vi "main_nova.vi"() -> ()   [LabVIEW 2020]
panel:
  out "Log":string
  in  "MoveJ 2":bool
  out "Error Log":string
  out "error out 3":errorcluster
  in  "MoveL":bool
  out "DigitalOutput":u8[](array[numeric])
  out "DigitalInput":u8[](array[numeric])
  out "Current SpeedFactor":dbl
  out "error out 2":errorcluster
  in  "Digital Outputs Index:":i32=1 min=1 max=16 step=1
  in  "GetErrorID":bool
  out "x value":string
  out "y value":string
  out "z value":string
  out "rx value":string
  out "ry value":string
  out "rz value":string
  out "j6 value":string
  out "j5 value":string
  out "j4 value":string
  out "j3 value":string
  out "j2 value":string
  out "j1 value":string
  in  "rz-":bool
  in  "ry-":bool
  in  "rx-":bool
  in  "z-":bool
  in  "y-":bool
  in  "x-":bool
  in  "rz+":bool
  in  "ry+":bool
  in  "rx+":bool
  in  "z+":bool
  in  "y+":bool
  in  "x+":bool
  in  "j6":dbl
  in  "j5":dbl
  in  "j4":dbl
  in  "j3":dbl
  in  "j2":dbl
  in  "j1":dbl
  in  "Set IO confrim":bool
  in  "Status":string(combo)="1"
  in  "Feedback Port":string="30004"
  in  "Dashboard Port":string="29999"
  in  "IP Address":string="192.168.5.1"
  in  "stop get state":bool
  out "state error out 2":errorcluster
  out "Robot mode":T1(ring)
  out "speed set string":string
  in  "j6-":bool
  in  "j5-":bool
  in  "j4-":bool
  in  "j3-":bool
  in  "j2-":bool
  in  "j1-":bool
  in  "j6+":bool
  in  "j5+":bool
  in  "j4+":bool
  in  "j3+":bool
  in  "j2+":bool
  in  "j1+":bool
  in  "stop connect":bool
  in  "Start trace":bool
  in  "tracePath":string
  in  "Stop move":bool
  in  "MoveJ":bool
  in  "rz":dbl
  in  "ry":dbl
  in  "rx":dbl
  in  "z":dbl
  in  "y":dbl
  in  "x":dbl
  in  "Speed confrim":bool
  in  "Speed Ratio":dbl=50.0
  in  "ClearError":bool
  in  "Enable Robot":bool
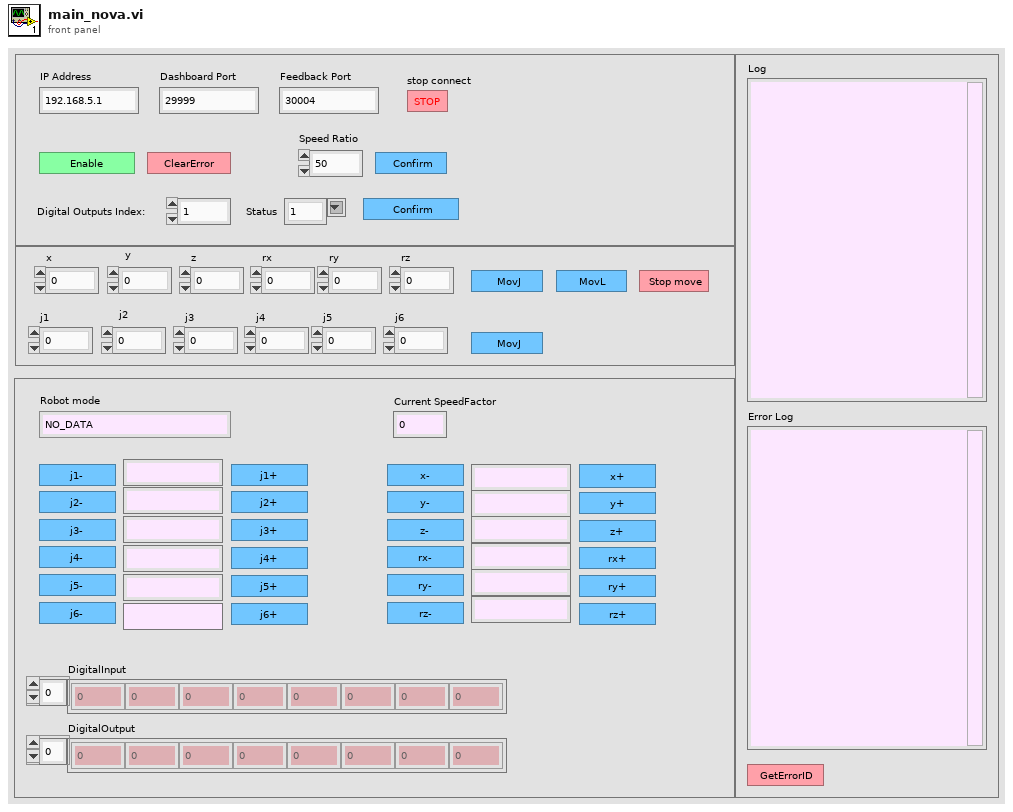
[diagram p1: front panel]
types:
  T1 = enum16{"NO_DATA", "ROBOT_MODE_INIT", "ROBOT_MODE_BRAKE_OPEN", "ROBOT_MODE_POWEROFF", "ROBOT_MODE_DISABLED", "ROBOT_MODE_ENABLE", "ROBOT_MODE_BACKDRIVE", "ROBOT_MODE_RUNNING", "ROBOT_MODE_SINGLE_MOVE", "ROBOT_MODE_ERROR", "ROBOT_MODE_PAUSE", "ROBOT_MODE_COLLISION"}
  T2 = enum16{"Standard", "Buffered", "CRLF", "Immediate"}
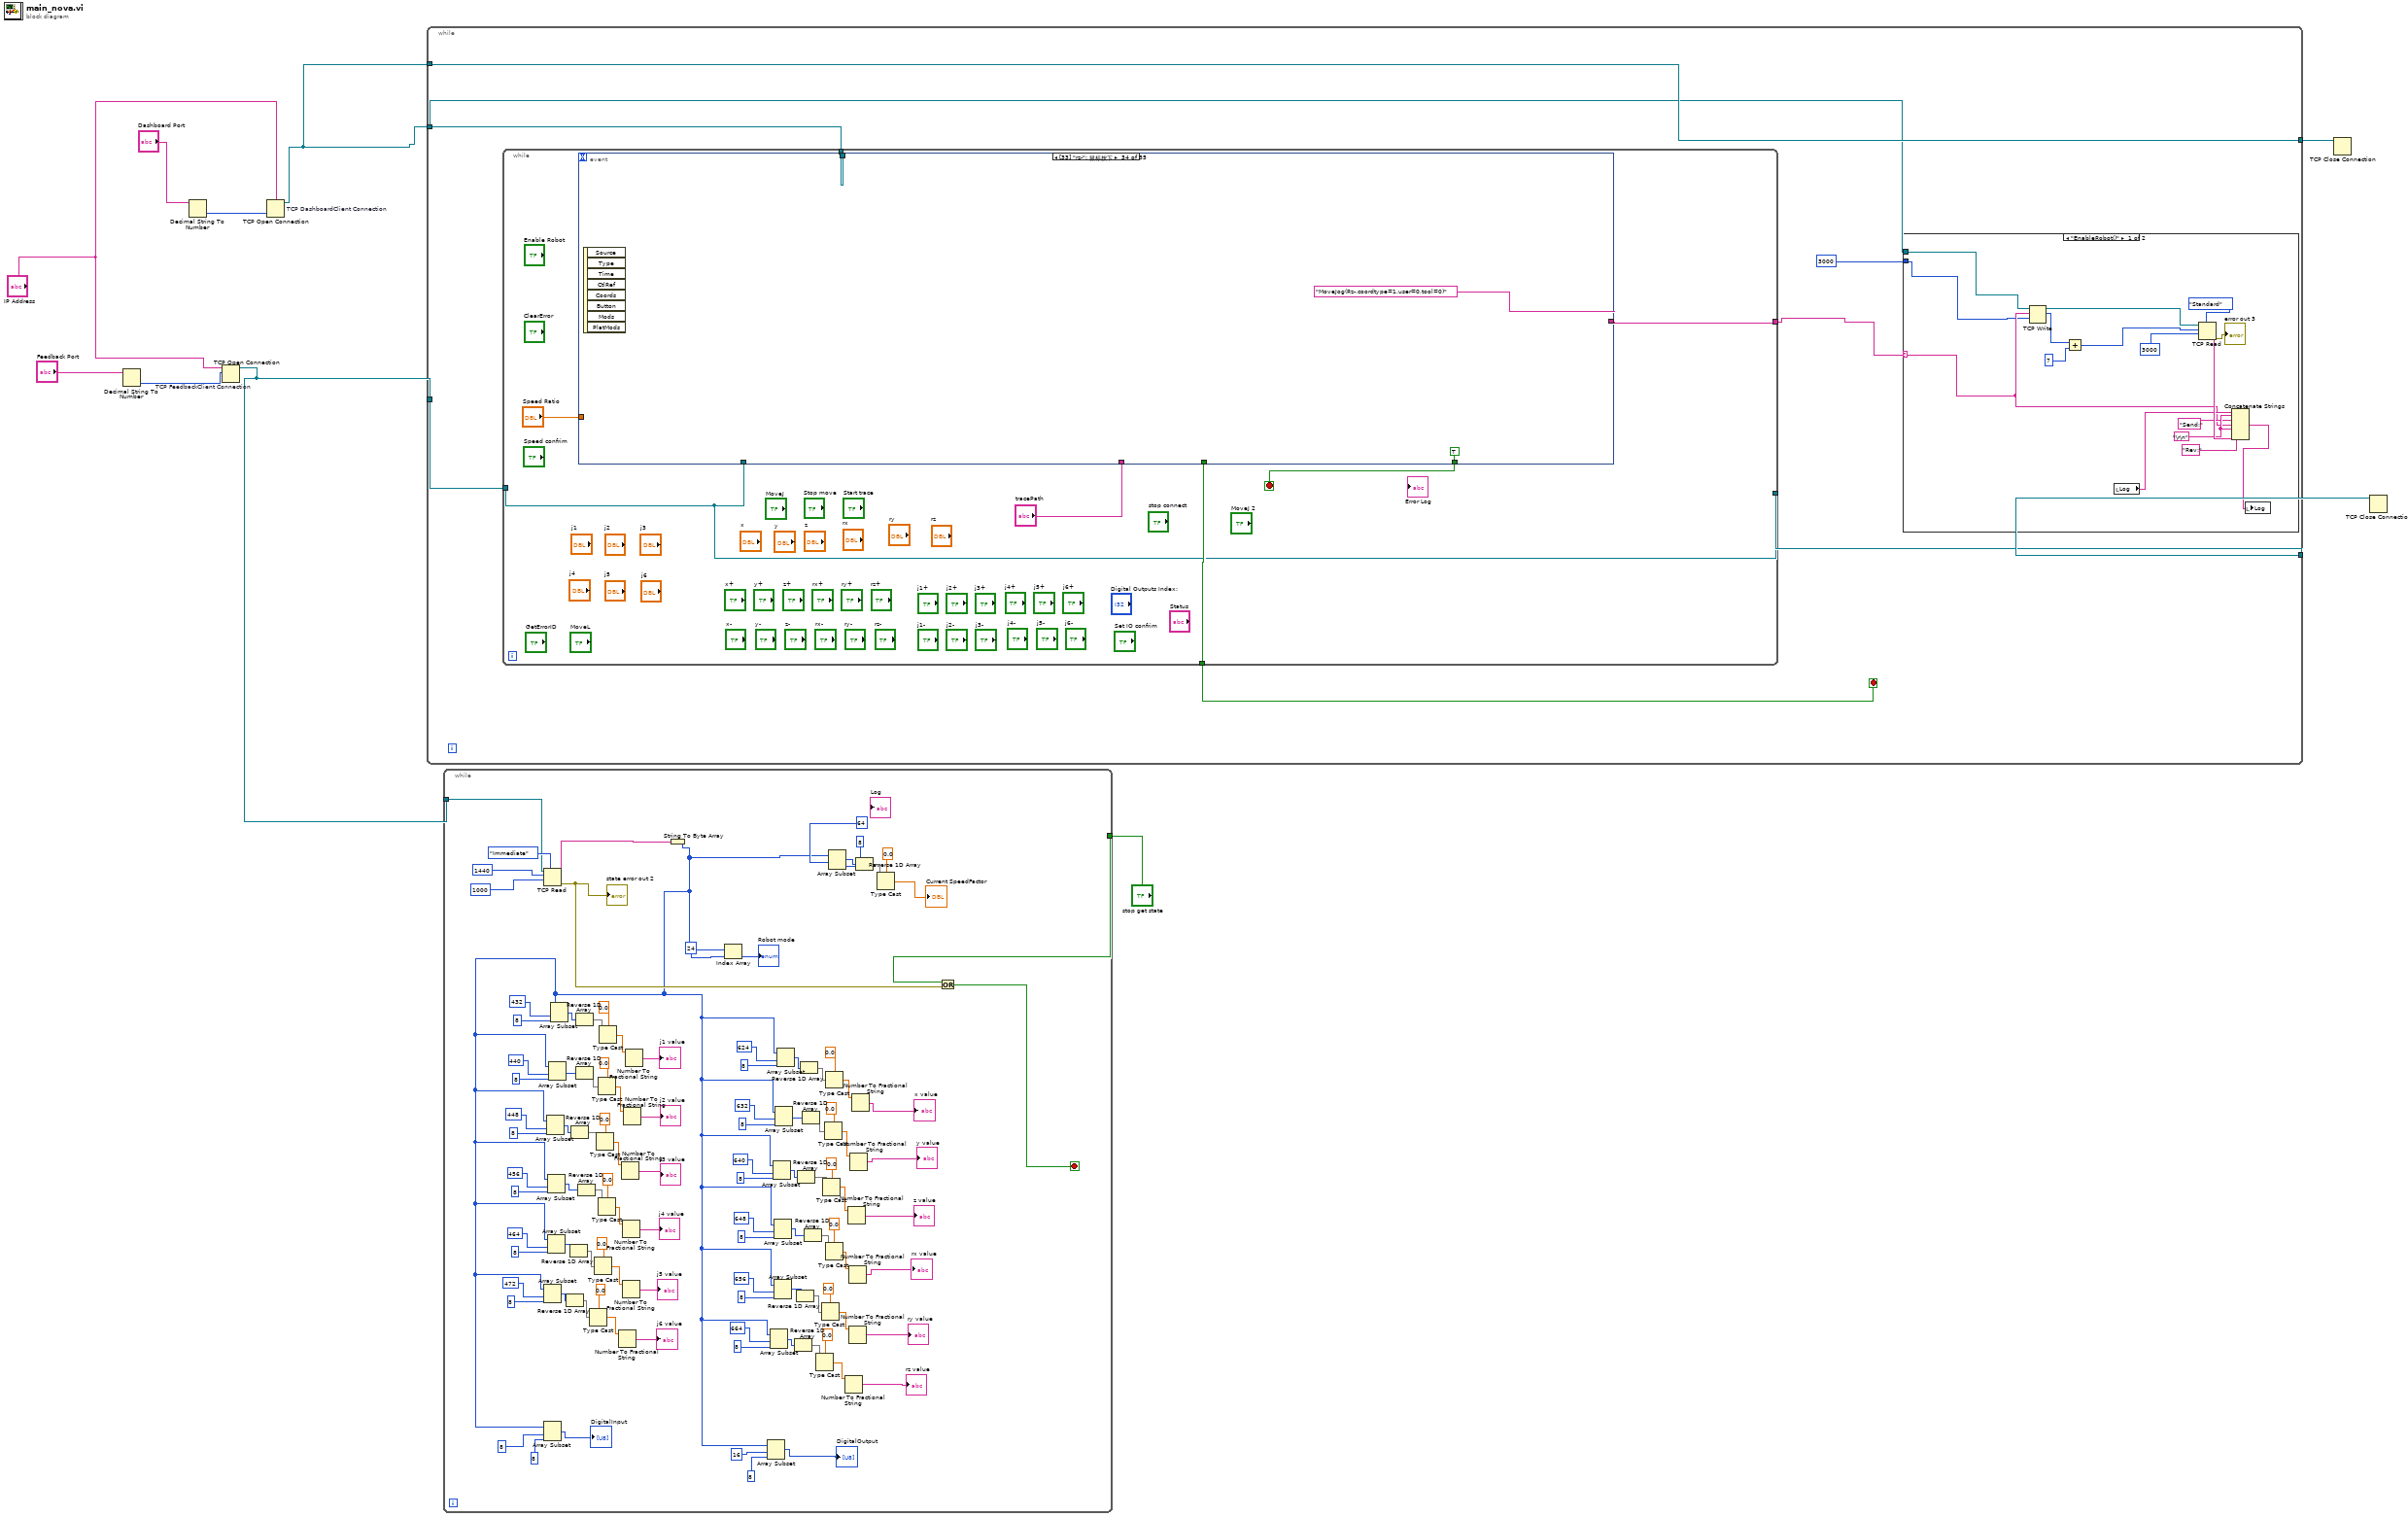
[diagram p0: block diagram]
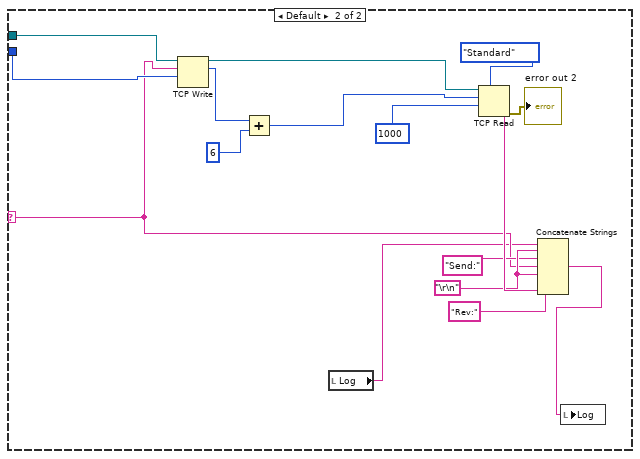
[diagram p2: hidden frame]
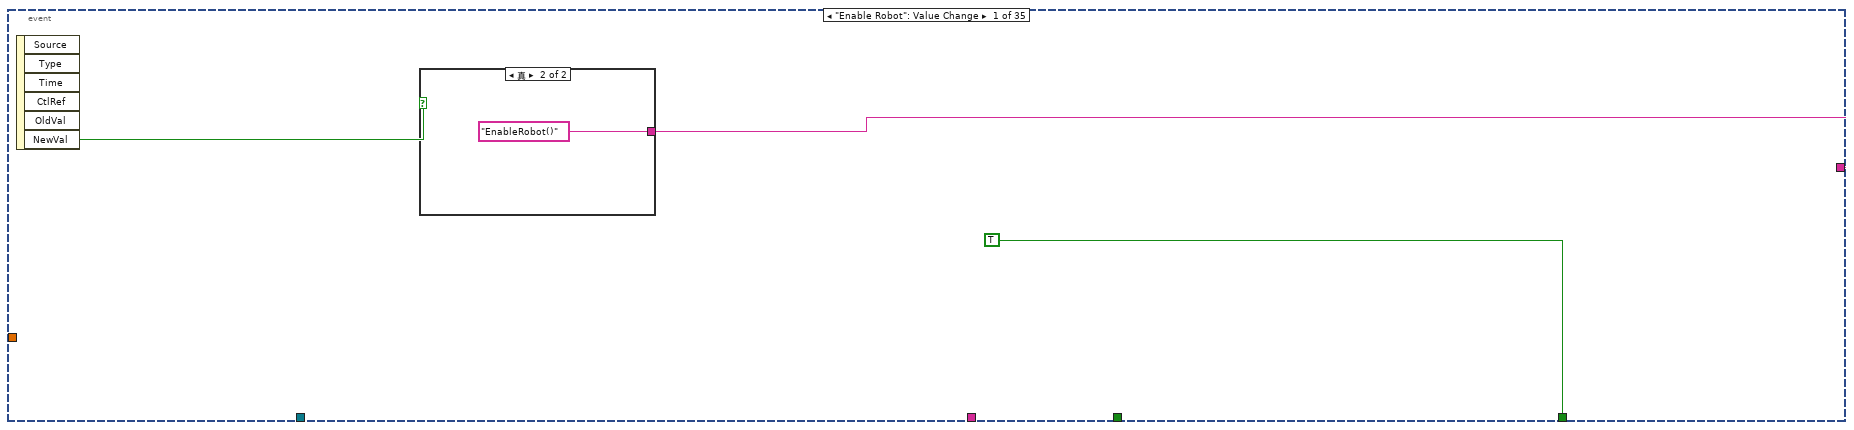
[diagram p3: hidden frame]
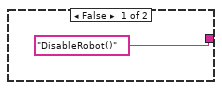
[diagram p4: hidden frame]
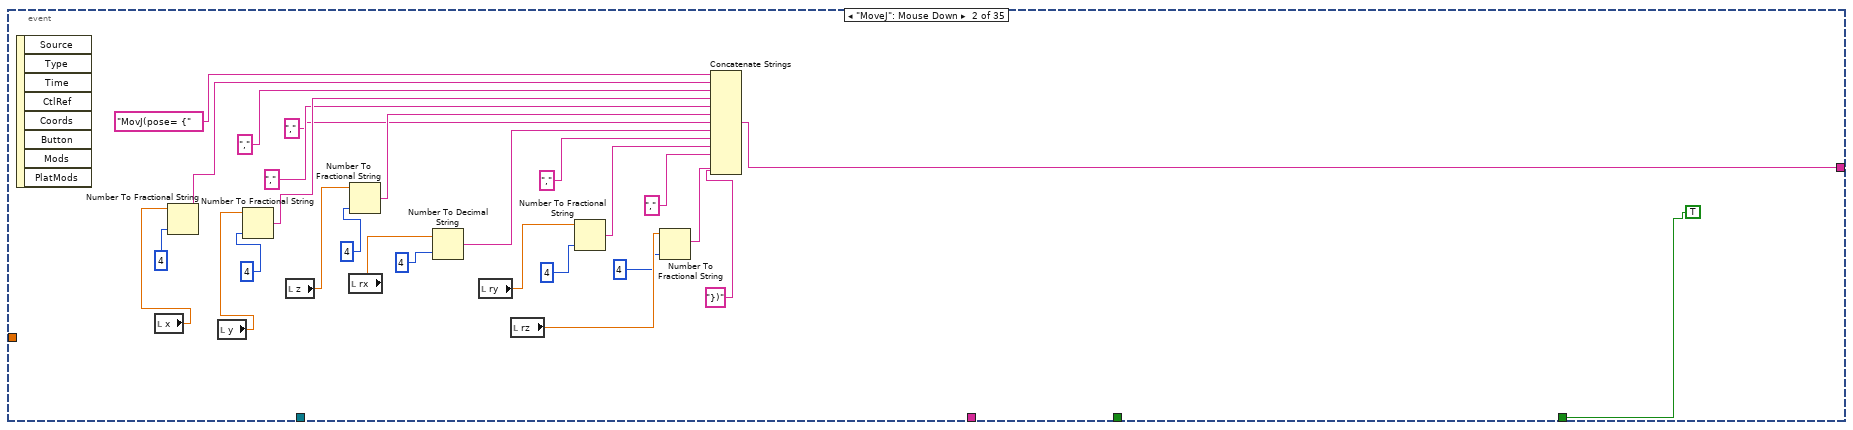
[diagram p5: hidden frame]
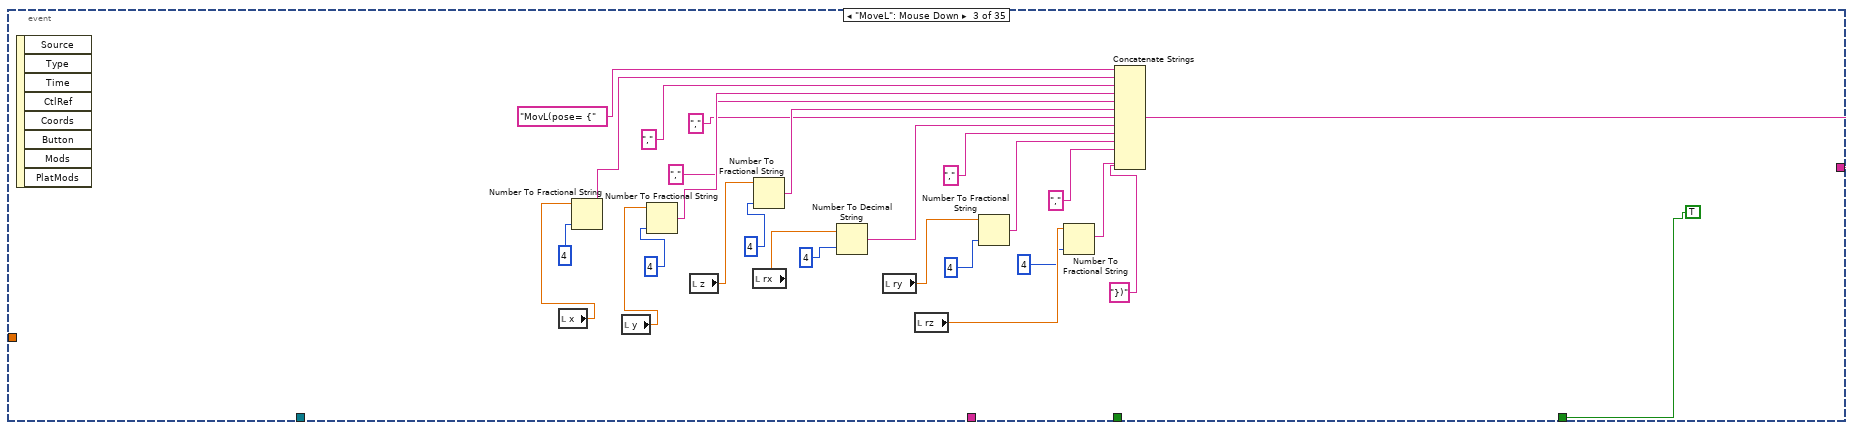
[diagram p6: hidden frame]
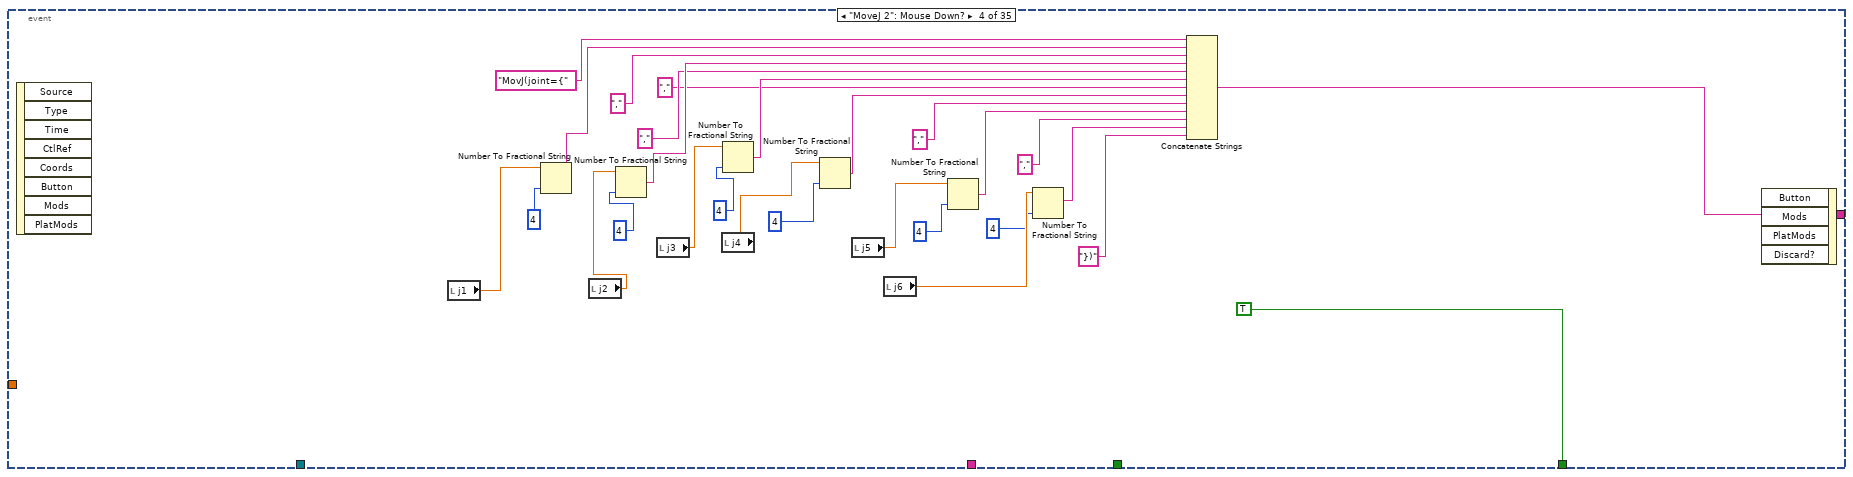
[diagram p7: hidden frame]
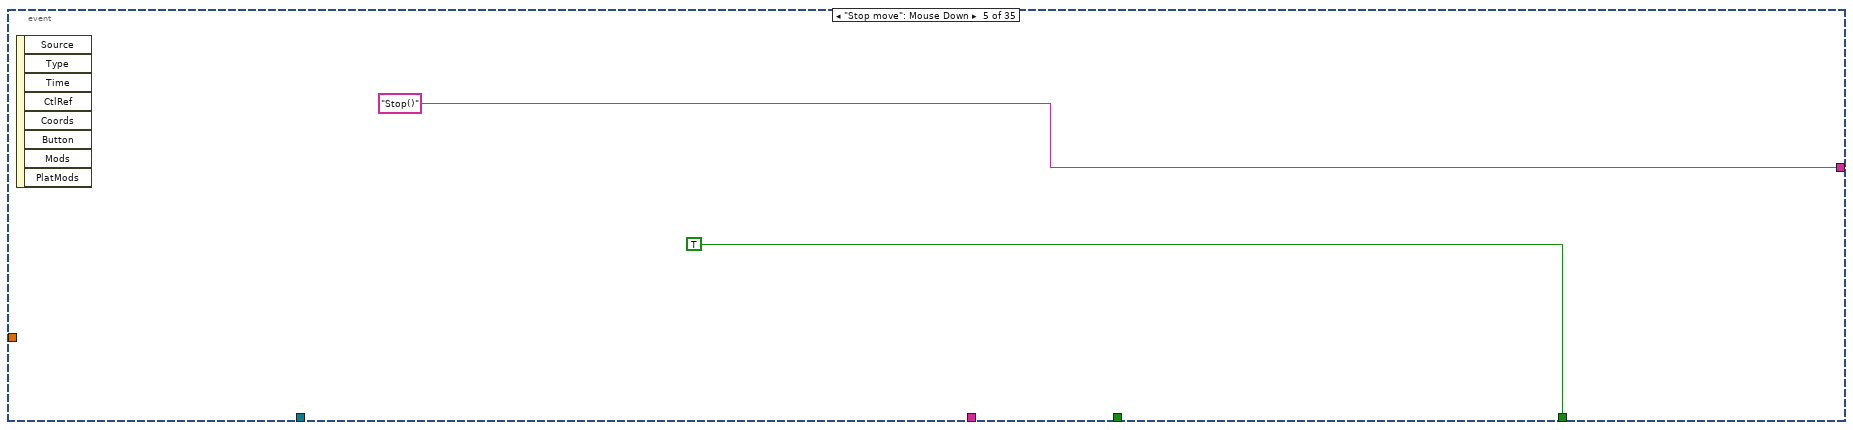
[diagram p8: hidden frame]
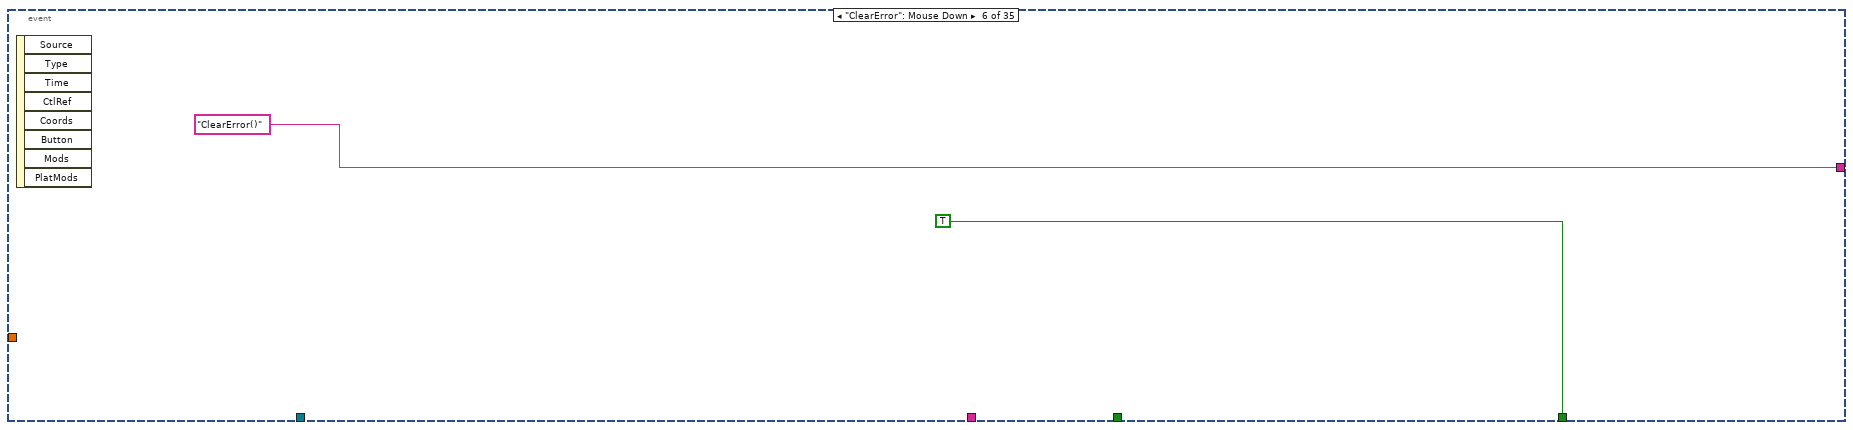
[diagram p9: hidden frame]
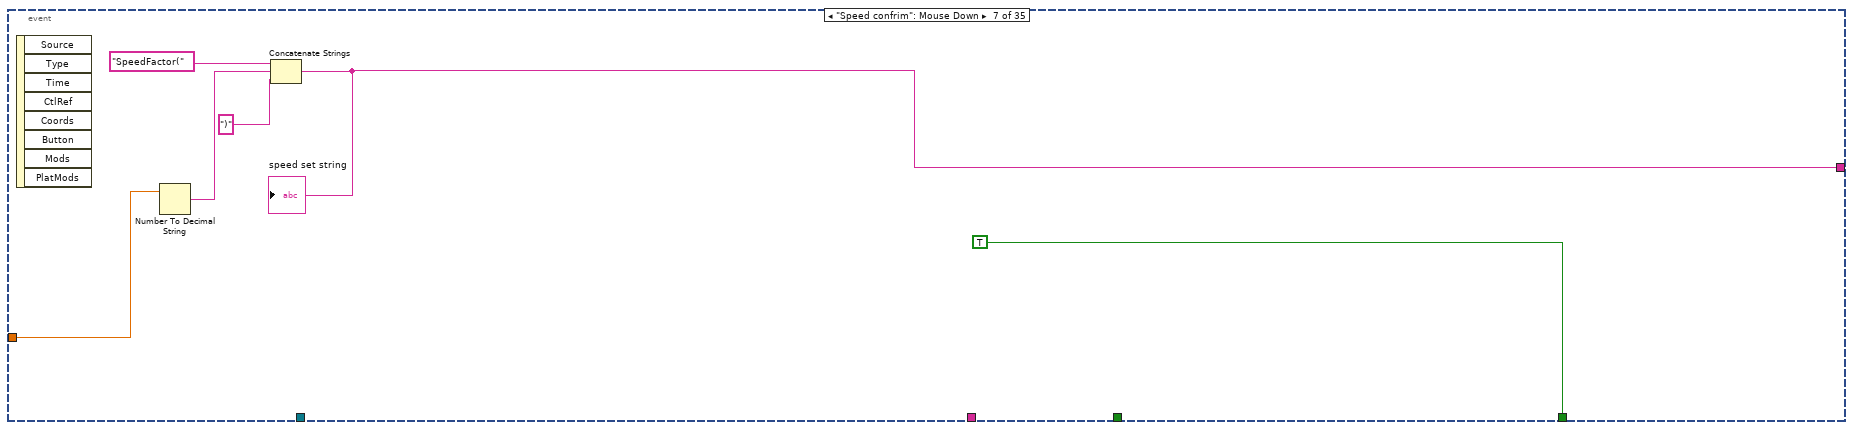
[diagram p10: hidden frame]
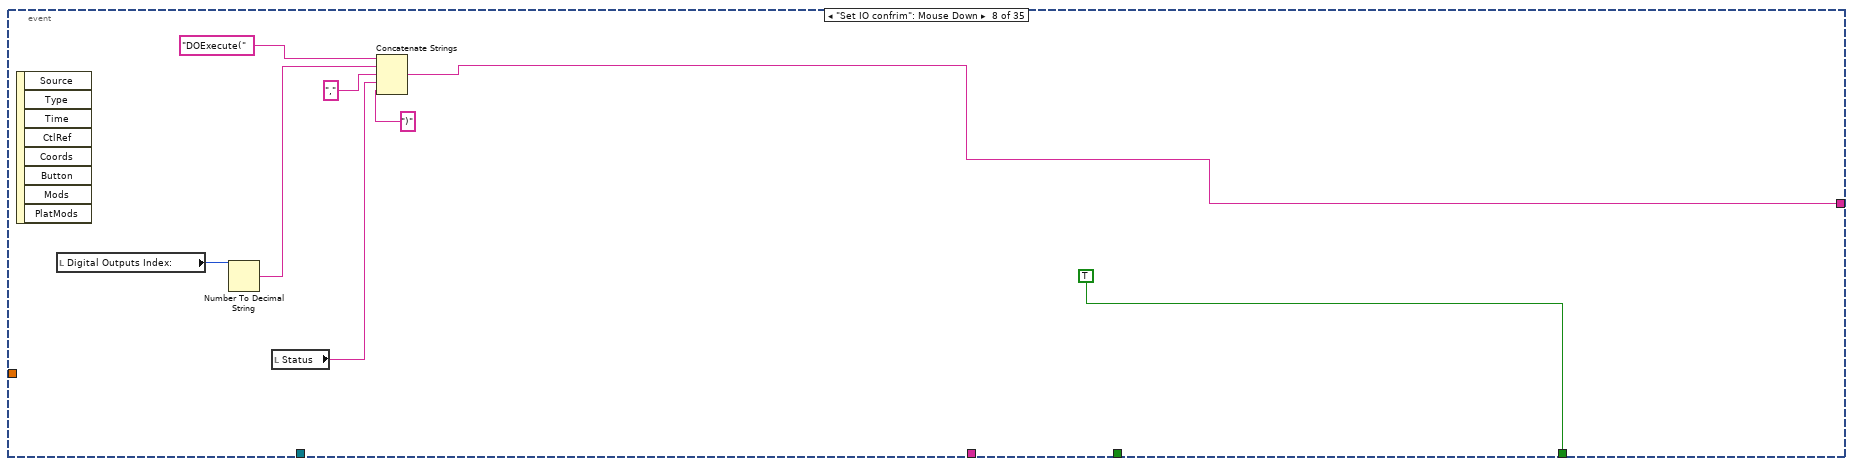
[diagram p11: hidden frame]
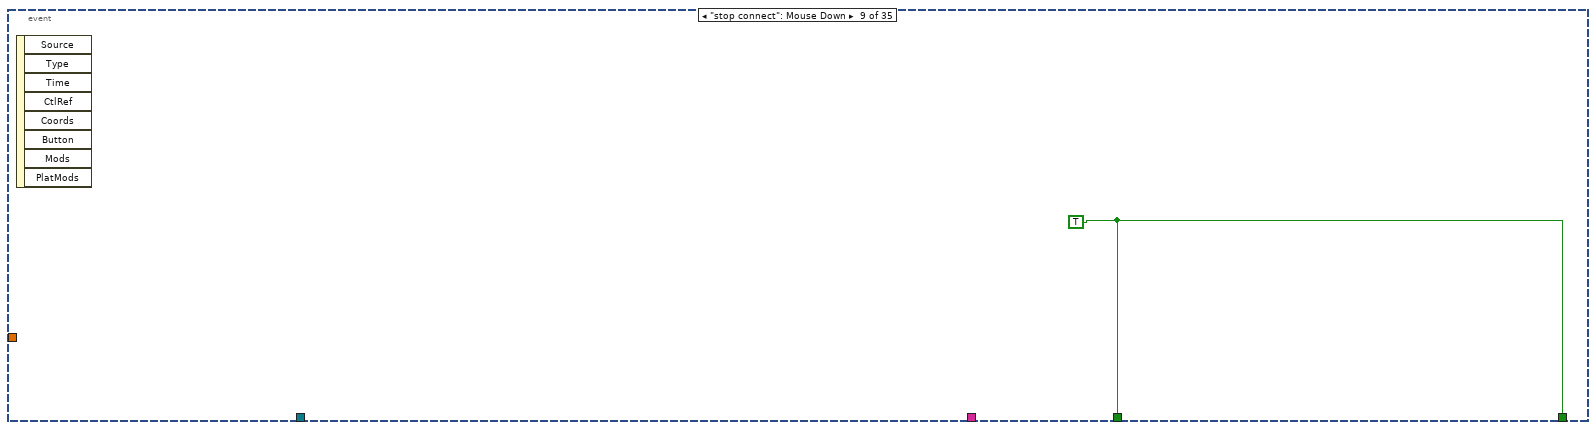
[diagram p12: hidden frame]
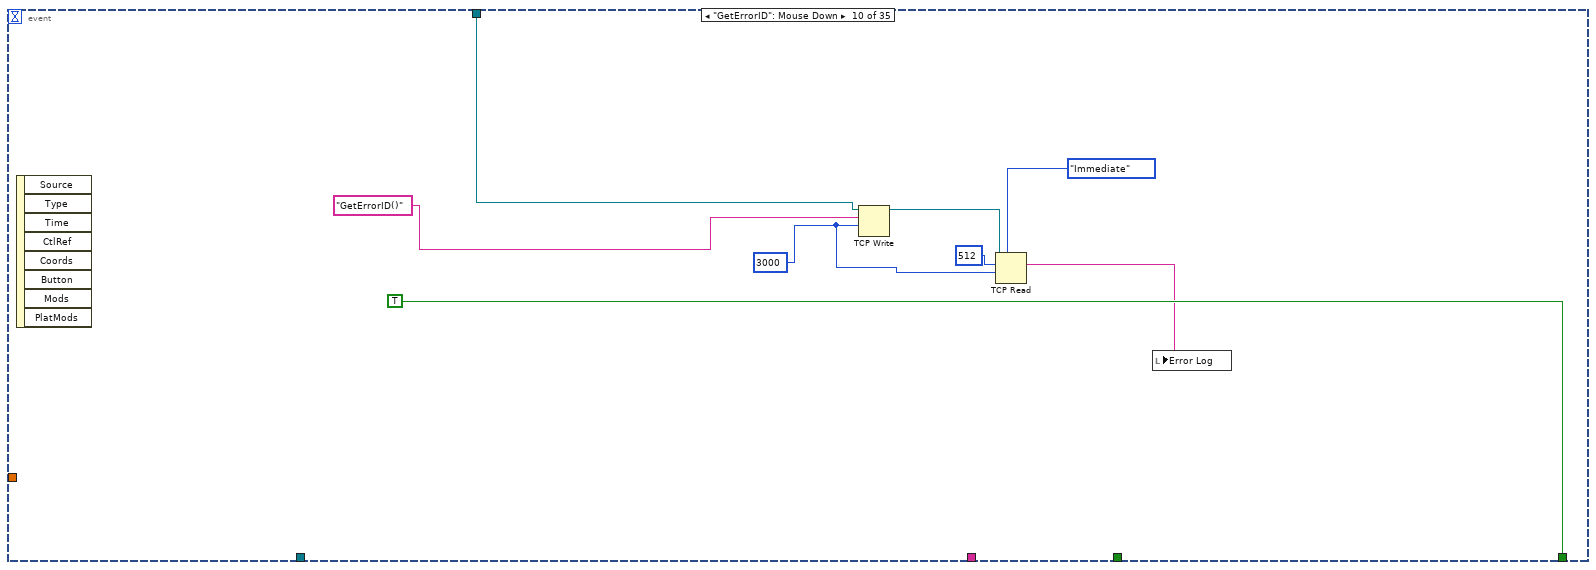
[diagram p13: hidden frame]
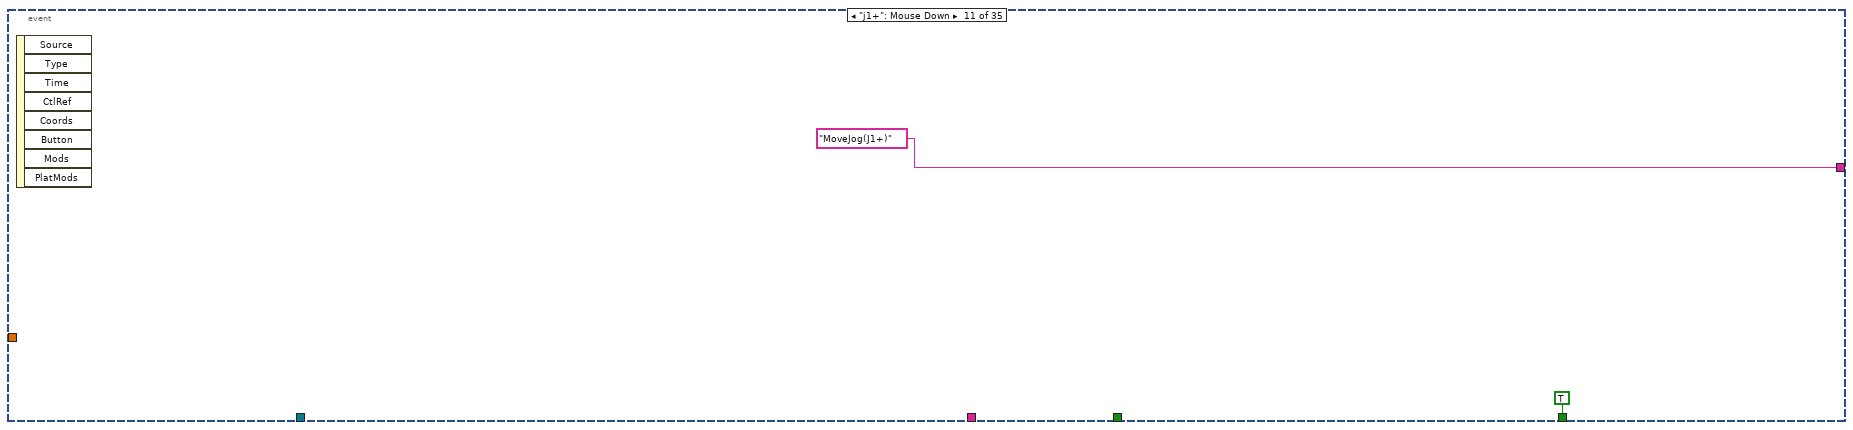
[diagram p14: hidden frame]
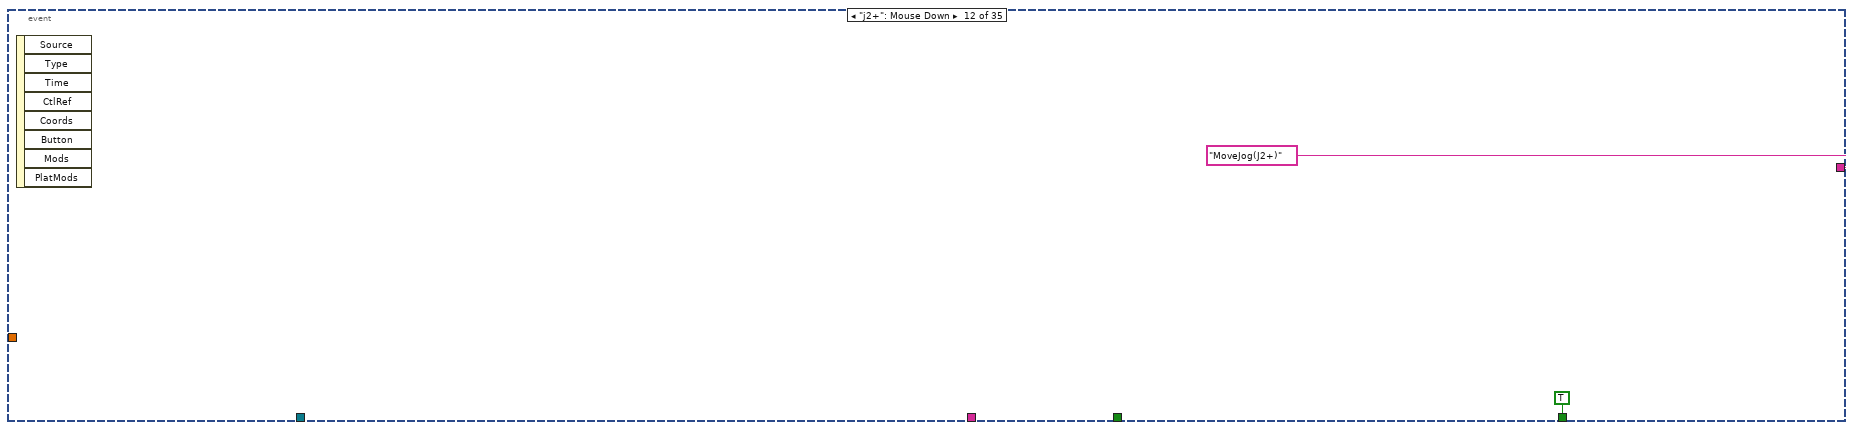
[diagram p15: hidden frame]
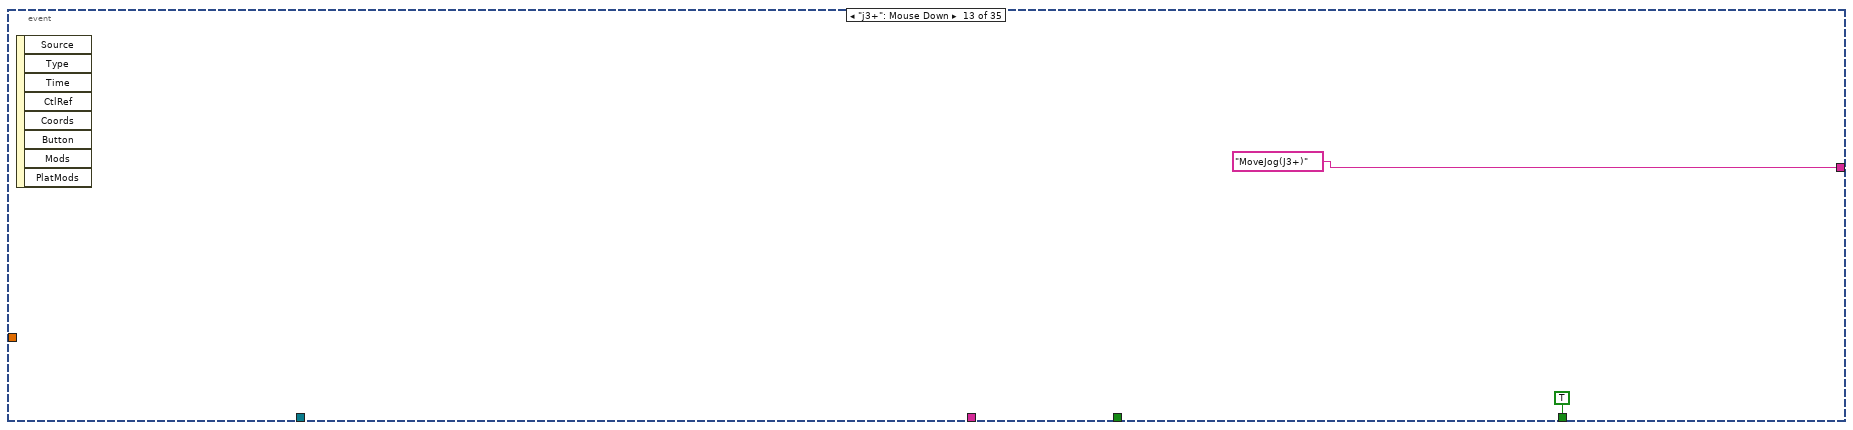
[diagram p16: hidden frame]
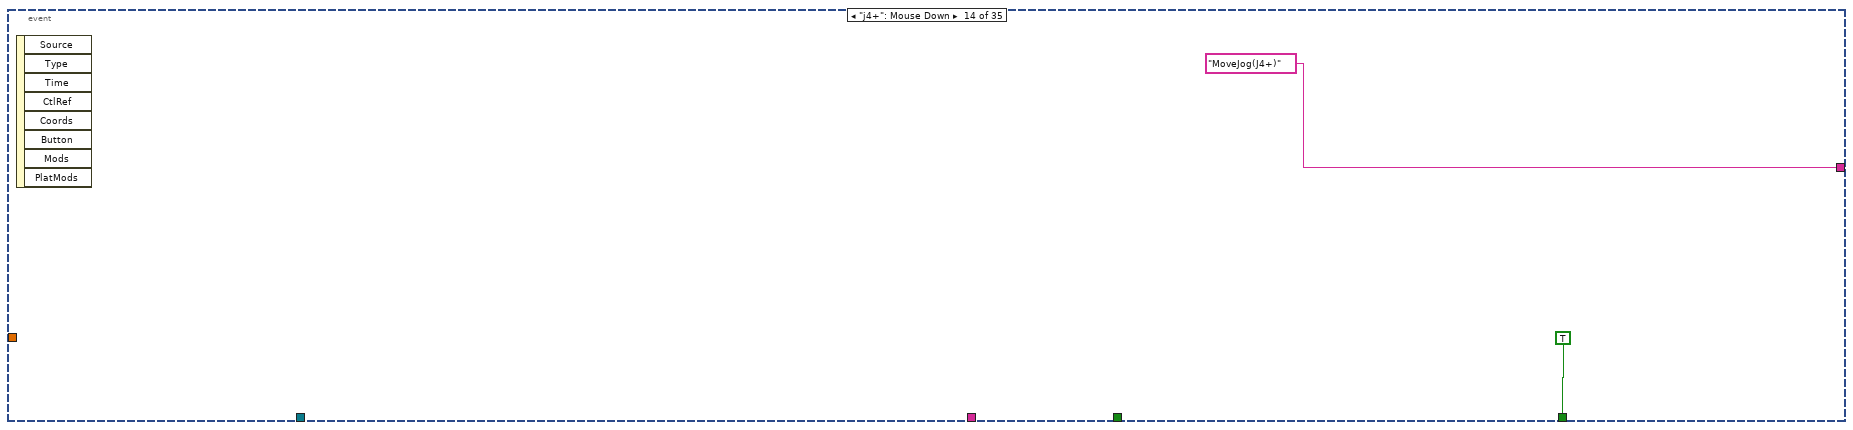
[diagram p17: hidden frame]
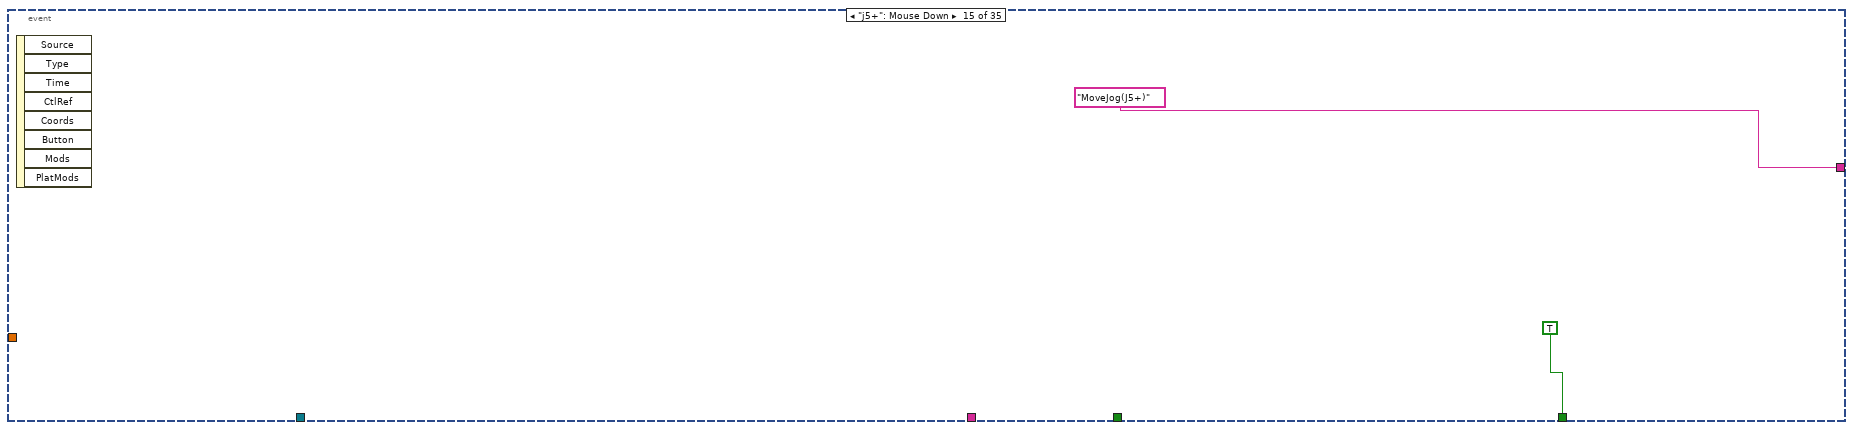
[diagram p18: hidden frame]
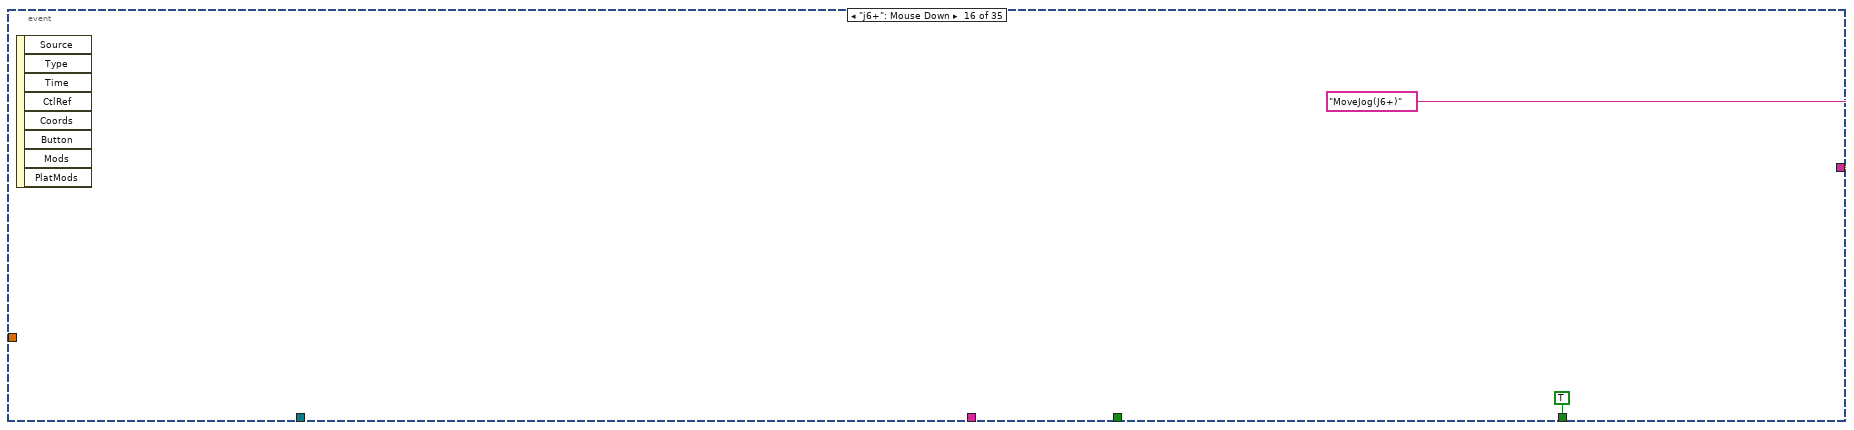
[diagram p19: hidden frame]
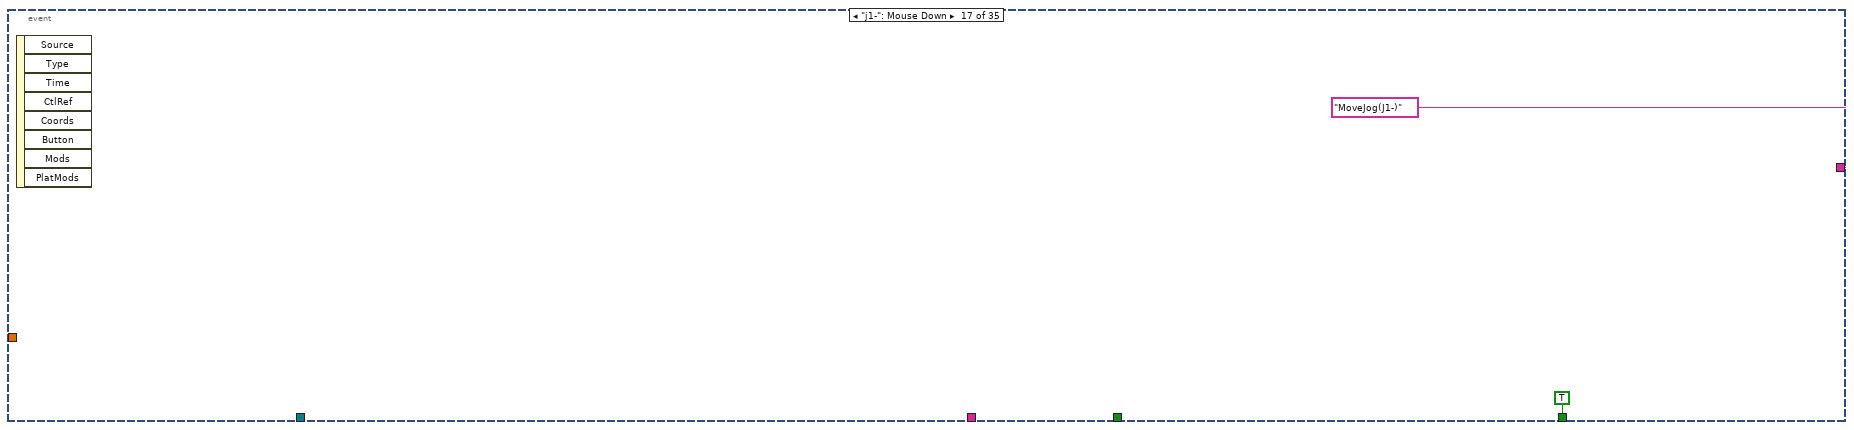
[diagram p20: hidden frame]
diagram:
  n1 = Decimal String To Number(string="Feedback Port") -> (number=w2:i32)  [unwired: 2 in, 1 out]
  n2 = Decimal String To Number(string="Dashboard Port") -> (number=w3:i32)  [unwired: 2 in, 1 out]
  n3 = TCP Open Connection "TCP FeedbackClient Connection"(address="IP Address", remote port or service name=w2) -> (connection ID=w7:refnum<k5>)  [unwired: 3 in, 1 out]
  n4 = TCP Open Connection "TCP DashboardClient Connection"(address="IP Address", remote port or service name=w3) -> (connection ID=w1:refnum<k5>)  [unwired: 3 in, 1 out]
  n5 = while {
    tunnel: [w17] -> w10
    tunnel: w1 -> [w17]
    tunnel: w7 -> [w15]
    tunnel: [w14] -> w9
    tunnel: w1 -> [w12]
    stop <- w16 stop-if-true
    n6 = while {
      tunnel: [w54] -> w16
      tunnel: w15 -> [w53]
      tunnel: [w53] -> w14
      tunnel: [w50] -> w13
      tunnel: w12 -> [w51]
      stop <- w55 stop-if-true
      n7 = event shown="[33] \"rz-\": 鼠标按下" {
        selector: _ -> [_ _ _ _ _ _ _ _ _ _ _ _ _ _ _ _ _ _ _ _ _ _ _ _ _ _ _ _ _ _ _ _ _ _ _]
        dyn-events: _ -> [_ _ _ _ _ _ _ _ _ _ _ _ _ _ _ _ _ _ _ _ _ _ _ _ _ _ _ _ _ _ _ _ _ _ _]
        timeout: _ -> [_ _ _ _ _ _ _ _ _ _ _ _ _ _ _ _ _ _ _ _ _ _ _ _ _ _ _ _ _ _ _ _ _ _ _]
        tunnel: [w57 w62 w89 w119 "Stop()" "ClearError()" w148 w156 _ _ "MoveJog(J1+)" "MoveJog(J2+)" "MoveJog(J3+)" "MoveJog(J4+)" "MoveJog(J5+)" "MoveJog(J6+)" "MoveJog(J1-)" "MoveJog(J2-)" "MoveJog(J3-)" "MoveJog(J4-)" "MoveJog(J5-)" "MoveJog(J6-)" "MoveJog(X+,coordtype=1,user=0,tool=0)" "MoveJog(Y+,coordtype=1,user=0,tool=0)" "MoveJog(Z+,coordtype=1,user=0,tool=0)" "MoveJog(Rx+,coordtype=1,user=0,tool=0)" "MoveJog(Ry+,coordtype=1,user=0,tool=0)" "MoveJog(Rz+,coordtype=1,user=0,tool=0)" "MoveJog(X-,coordtype=1,user=0,tool=0)" "MoveJog(Y-,coordtype=0,user=0,tool=0)" "MoveJog(Z-,coordtype=1,user=0,tool=0)" "MoveJog(Rx-,coordtype=1,user=0,tool=0)" "MoveJog(Ry-,coordtype=1,user=0,tool=0)" "MoveJog(Rz-,coordtype=1,user=0,tool=0)" "MoveJog()"] -> w50
        tunnel: "tracePath" -> [_ _ _ _ _ _ _ _ _ _ _ _ _ _ _ _ _ _ _ _ _ _ _ _ _ _ _ _ _ _ _ _ _ _ _]
        tunnel: [TRUE TRUE TRUE TRUE TRUE TRUE TRUE TRUE w161 TRUE TRUE TRUE TRUE TRUE TRUE TRUE TRUE TRUE TRUE TRUE TRUE TRUE TRUE TRUE TRUE TRUE TRUE TRUE TRUE TRUE TRUE TRUE TRUE TRUE TRUE] -> w55
        tunnel: [_ _ _ _ _ _ _ _ w161 _ _ _ _ _ _ _ _ _ _ _ _ _ _ _ _ _ _ _ _ _ _ _ _ _ _] -> w54
        tunnel: w53 -> [_ _ _ _ _ _ _ _ _ _ _ _ _ _ _ _ _ _ _ _ _ _ _ _ _ _ _ _ _ _ _ _ _ _ _]
        tunnel: "Speed Ratio" -> [_ _ _ _ _ _ w147 _ _ _ _ _ _ _ _ _ _ _ _ _ _ _ _ _ _ _ _ _ _ _ _ _ _ _ _]
        tunnel: w51 -> [_ _ _ _ _ _ _ _ _ w163 _ _ _ _ _ _ _ _ _ _ _ _ _ _ _ _ _ _ _ _ _ _ _ _ _]
        event "Enable Robot": Value Change {
          n8 = event-data() -> ("NewVal"=w59:bool)  [unwired: 1 in, 5 out]
          n9 = case shown="真" w59 {
            tunnel: ["DisableRobot()" "EnableRobot()"] -> w57
            frame False {
            }
            frame True {
            }
          }
        }
        event "MoveJ": Mouse Down {
          n10 = event-data() -> ()  [unwired: 1 in, 8 out]
          n11 = local read "x"() -> (w63:dbl)
          n12 = Number To Fractional String(number=w63, precision (6)=i16 4) -> (F-format string=w77:string)  [unwired: 2 in]
          n13 = local read "y"() -> (w87:dbl)
          n14 = Number To Fractional String(number=w87, precision (6)=i16 4) -> (F-format string=w78:string)  [unwired: 2 in]
          n15 = local read "z"() -> (w86:dbl)
          n16 = local read "rx"() -> (w85:dbl)
          n17 = Number To Fractional String(number=w86, precision (6)=i16 4) -> (F-format string=w82:string)  [unwired: 2 in]
          n18 = Number To Decimal String(number=w85, width (-)=i16 4 ("precision (6)")) -> (decimal integer string=w79:string)
          n19 = local read "ry"() -> (w84:dbl)
          n20 = local read "rz"() -> (w83:dbl)
          n21 = Number To Fractional String(number=w84, precision (6)=i16 4) -> (F-format string=w80:string)  [unwired: 2 in]
          n22 = Number To Fractional String(number=w83, precision (6)=i16 4) -> (F-format string=w81:string)  [unwired: 2 in]
          n23 = Concatenate Strings("MovJ(pose= {" ("string"), w77, "," ("string"), w78, "," ("string"), w82, "," ("string"), w79, "," ("string"), w80, "," ("string"), w81, "})" ("string")) -> (w62:string)
        }
        event "MoveL": Mouse Down {
          n24 = event-data() -> ()  [unwired: 1 in, 8 out]
          n25 = local read "x"() -> (w114:dbl)
          n26 = Number To Fractional String(number=w114, precision (6)=i16 4) -> (F-format string=w103:string)  [unwired: 2 in]
          n27 = local read "y"() -> (w113:dbl)
          n28 = Number To Fractional String(number=w113, precision (6)=i16 4) -> (F-format string=w104:string)  [unwired: 2 in]
          n29 = local read "z"() -> (w112:dbl)
          n30 = local read "rx"() -> (w111:dbl)
          n31 = Number To Fractional String(number=w112, precision (6)=i16 4) -> (F-format string=w108:string)  [unwired: 2 in]
          n32 = Number To Decimal String(number=w111, width (-)=i16 4 ("precision (6)")) -> (decimal integer string=w105:string)
          n33 = local read "ry"() -> (w110:dbl)
          n34 = local read "rz"() -> (w109:dbl)
          n35 = Number To Fractional String(number=w110, precision (6)=i16 4) -> (F-format string=w106:string)  [unwired: 2 in]
          n36 = Number To Fractional String(number=w109, precision (6)=i16 4) -> (F-format string=w107:string)  [unwired: 2 in]
          n37 = Concatenate Strings("MovL(pose= {" ("string"), w103, "," ("string"), w104, "," ("string"), w108, "," ("string"), w105, "," ("string"), w106, "," ("string"), w107, "})" ("string")) -> (w89:string)
        }
        event "MoveJ 2": Mouse Down? {
          n38 = event-data() -> ()  [unwired: 1 in, 8 out]
          n39 = local read "j1"() -> (w121:dbl)
          n40 = Number To Fractional String(number=w121, precision (6)=i16 4) -> (F-format string=w134:string)  [unwired: 2 in]
          n41 = local read "j2"() -> (w142:dbl)
          n42 = Number To Fractional String(number=w142, precision (6)=i16 4) -> (F-format string=w135:string)  [unwired: 2 in]
          n43 = local read "j3"() -> (w141:dbl)
          n44 = local read "j4"() -> (w117:dbl)
          n45 = Number To Fractional String(number=w141, precision (6)=i16 4) -> (F-format string=w138:string)  [unwired: 2 in]
          n46 = Number To Fractional String(number=w117, precision (6)=i16 4) -> (F-format string=w116:string)  [unwired: 2 in]
          n47 = local read "j5"() -> (w140:dbl)
          n48 = local read "j6"() -> (w139:dbl)
          n49 = Number To Fractional String(number=w140, precision (6)=i16 4) -> (F-format string=w136:string)  [unwired: 2 in]
          n50 = Number To Fractional String(number=w139, precision (6)=i16 4) -> (F-format string=w137:string)  [unwired: 2 in]
          n51 = Concatenate Strings("MovJ(joint={" ("string"), w134, "," ("string"), w135, "," ("string"), w138, "," ("string"), w116, "," ("string"), w136, "," ("string"), w137, "})" ("string")) -> (w119:string)
          n52 = event-data() -> ()  [unwired: 5 in, 1 out]
        }
        event "Stop move": Mouse Down {
          n53 = event-data() -> ()  [unwired: 1 in, 8 out]
        }
        event "ClearError": Mouse Down {
          n54 = event-data() -> ()  [unwired: 1 in, 8 out]
        }
        event "Speed confrim": Mouse Down {
          n55 = event-data() -> ()  [unwired: 1 in, 8 out]
          n56 = Number To Decimal String(number=w147) -> (decimal integer string=w152:string)  [unwired: 1 in]
          n57 = Concatenate Strings("SpeedFactor(", w152, ")") -> (w148:string)
          "speed set string" <- w148
        }
        event "Set IO confrim": Mouse Down {
          n58 = event-data() -> ()  [unwired: 1 in, 8 out]
          n59 = local read "Digital Outputs Index:"() -> (w154:i32)
          n60 = Number To Decimal String(number=w154) -> (decimal integer string=w160:string)  [unwired: 1 in]
          n61 = local read "Status"() -> (w153:string)
          n62 = Concatenate Strings("DOExecute(", w160, "," ("string"), w153, ")") -> (w156:string)
        }
        event "stop connect": Mouse Down {
          w161 = TRUE
          n63 = event-data() -> ()  [unwired: 1 in, 8 out]
        }
        event "GetErrorID": Mouse Down {
          w166 = 3000 ("timeout ms (25000)")
          n64 = event-data() -> ()  [unwired: 1 in, 8 out]
          n65 = TCP Write(connection ID=w163, data in="GetErrorID()", 9:w166) -> (connection ID out=w167:refnum<k5>)  [unwired: 1 in, 2 out]
          n66 = TCP Read(connection ID=w167, bytes to read=512, 7:T2."Immediate" ("mode (standard)"), 9:w166) -> (data out=w162:string)  [unwired: 1 in, 2 out]
          n67 = local write "Error Log"(w162) -> ()
        }
        event "j1+": Mouse Down {
          n68 = event-data() -> ()  [unwired: 1 in, 8 out]
        }
        event "j2+": Mouse Down {
          n69 = event-data() -> ()  [unwired: 1 in, 8 out]
        }
        event "j3+": Mouse Down {
          n70 = event-data() -> ()  [unwired: 1 in, 8 out]
        }
        event "j4+": Mouse Down {
          n71 = event-data() -> ()  [unwired: 1 in, 8 out]
        }
        event "j5+": Mouse Down {
          n72 = event-data() -> ()  [unwired: 1 in, 8 out]
        }
        event "j6+": Mouse Down {
          n73 = event-data() -> ()  [unwired: 1 in, 8 out]
        }
        event "j1-": Mouse Down {
          n74 = event-data() -> ()  [unwired: 1 in, 8 out]
        }
        event "j2-": Mouse Down {
          n75 = event-data() -> ()  [unwired: 1 in, 8 out]
        }
        event "j3-": Mouse Down {
          n76 = event-data() -> ()  [unwired: 1 in, 8 out]
        }
        event "j4-": Mouse Down {
          n77 = event-data() -> ()  [unwired: 1 in, 8 out]
        }
        event "j5-": Mouse Down {
          n78 = event-data() -> ()  [unwired: 1 in, 8 out]
        }
        event "j6-": Mouse Down {
          n79 = event-data() -> ()  [unwired: 1 in, 8 out]
        }
        event "x+": Mouse Down {
          n80 = event-data() -> ()  [unwired: 1 in, 8 out]
        }
        event "y+": Mouse Down {
          n81 = event-data() -> ()  [unwired: 1 in, 8 out]
        }
        event "z+": Mouse Down {
          n82 = event-data() -> ()  [unwired: 1 in, 8 out]
        }
        event "rx+": Mouse Down {
          n83 = event-data() -> ()  [unwired: 1 in, 8 out]
        }
        event "ry+": Mouse Down {
          n84 = event-data() -> ()  [unwired: 1 in, 8 out]
        }
        event "rz+": Mouse Down {
          n85 = event-data() -> ()  [unwired: 1 in, 8 out]
        }
        event "x-": Mouse Down {
          n86 = event-data() -> ()  [unwired: 1 in, 8 out]
        }
        event "y-": Mouse Down {
          n87 = event-data() -> ()  [unwired: 1 in, 8 out]
        }
        event "z-": Mouse Down {
          n88 = event-data() -> ()  [unwired: 1 in, 8 out]
        }
        event "rx-": Mouse Down {
          n89 = event-data() -> ()  [unwired: 1 in, 8 out]
        }
        event "ry-": Mouse Down {
          n90 = event-data() -> ()  [unwired: 1 in, 8 out]
        }
        event "rz-": Mouse Down {
          n91 = event-data() -> ()  [unwired: 1 in, 8 out]
        }
        event "j6-", "j2+", "j3+", "j4+", "j5+", "j6+", "j1-", "j2-", "j3-", "j4-", "j5-", "x+", "y+", "z+", "rx+", "ry+", "rz+", "x-", "y-", "z-", "rx-", "ry-", "rz-", "j1+": Mouse Up {
          n92 = event-data() -> ()  [unwired: 1 in, 8 out]
        }
      }
    }
    n93 = case shown="\"EnableRobot()\"" w13 {
      tunnel: 3000 ("timeout ms (25000)") -> [w19 w41]
      tunnel: w12 -> [w18 w40]
      selector: w13 -> [w20 w39]
      frame "EnableRobot()" {
        w30 = "\r\n"
        n94 = TCP Write(connection ID=w18, data in=w20, 9:w19) -> (connection ID out=w31:refnum<k5>, bytes written=w23:i32)  [unwired: 1 in, 1 out]
        n95 = Add(x=w23, y=7) -> (x+y=w22:i32)
        n96 = local read "Log"() -> (w24:string)
        n97 = TCP Read(connection ID=w31, bytes to read=w22, 7:T2."Standard" ("mode (standard)"), 9:3000 ("timeout ms (25000)")) -> (data out=w32:string, error out=→"error out 3":errorcluster)  [unwired: 1 in, 1 out]
        n98 = Concatenate Strings(w24, w30, "Send:" ("string"), w20, w30, "Rev:" ("string"), w32) -> (w25:string)
        n99 = local write "Log"(w25) -> ()
      }
      frame Default {
        w46 = "\r\n"
        n100 = TCP Write(connection ID=w40, data in=w39, 9:w41) -> (connection ID out=w47:refnum<k5>, bytes written=w36:i32)  [unwired: 1 in, 1 out]
        n101 = Add(x=w36, y=6) -> (x+y=w35:i32)
        n102 = local read "Log"() -> (w37:string)
        n103 = TCP Read(connection ID=w47, bytes to read=w35, 7:T2."Standard" ("mode (standard)"), 9:1000 ("timeout ms (25000)")) -> (data out=w48:string, error out=→"error out 2":errorcluster)  [unwired: 1 in, 1 out]
        n104 = Concatenate Strings(w37, w46, "Send:" ("string"), w39, w46, "Rev:" ("string"), w48) -> (w38:string)
        n105 = local write "Log"(w38) -> ()
      }
    }
  }
  n106 = while {
    tunnel: w7 -> [w323]
    tunnel: "stop get state" -> [w320]
    stop <- w319 stop-if-true
    n107 = TCP Read(connection ID=w323, bytes to read=1440, 7:T2."Immediate" ("mode (standard)"), 9:1000 ("timeout ms (25000)")) -> (data out=w321:string, error out=w318:errorcluster)  [unwired: 1 in, 1 out]
    "state error out 2" <- w318
    n108 = String To Byte Array(string=w321) -> (unsigned byte array=w222:u8[])
    n109 = Array Subset(array=w222, index=472, length=8) -> (w237:u8[])
    n110 = Array Subset(array=w222, index=8, length=8) -> (→"DigitalInput":u8[])
    n111 = Array Subset(array=w222, index=448, length=8) -> (w283:u8[])
    n112 = Array Subset(array=w222, index=456, length=8) -> (w281:u8[])
    n113 = Array Subset(array=w222, index=464, length=8) -> (w279:u8[])
    n114 = Array Subset(array=w222, index=440, length=8) -> (w284:u8[])
    n115 = Array Subset(array=w222, index=432, length=8) -> (w287:u8[])
    n116 = Reverse 1D Array(array=w237) -> (reversed array=w236:u8[])
    n117 = Reverse 1D Array(array=w279) -> (reversed array=w278:u8[])
    n118 = Reverse 1D Array(array=w283) -> (reversed array=w282:u8[])
    n119 = Reverse 1D Array(array=w287) -> (reversed array=w286:u8[])
    n120 = Reverse 1D Array(array=w284) -> (reversed array=w285:u8[])
    n121 = Reverse 1D Array(array=w281) -> (reversed array=w280:u8[])
    n122 = Type Cast(type=0.0, x=w236) -> (*(type *) &x=w292:dbl)
    n123 = Type Cast(type=0.0, x=w278) -> (*(type *) &x=w296:dbl)
    n124 = Type Cast(type=0.0, x=w282) -> (*(type *) &x=w304:dbl)
    n125 = Type Cast(type=0.0, x=w285) -> (*(type *) &x=w309:dbl)
    n126 = Type Cast(type=0.0, x=w280) -> (*(type *) &x=w300:dbl)
    n127 = Type Cast(type=0.0, x=w286) -> (*(type *) &x=w314:dbl)
    n128 = Number To Fractional String(number=w292) -> (F-format string=→"j6 value":string)  [unwired: 3 in]
    n129 = Number To Fractional String(number=w304) -> (F-format string=→"j3 value":string)  [unwired: 3 in]
    n130 = Number To Fractional String(number=w300) -> (F-format string=→"j4 value":string)  [unwired: 3 in]
    n131 = Number To Fractional String(number=w296) -> (F-format string=→"j5 value":string)  [unwired: 3 in]
    n132 = Number To Fractional String(number=w309) -> (F-format string=→"j2 value":string)  [unwired: 3 in]
    n133 = Number To Fractional String(number=w314) -> (F-format string=→"j1 value":string)  [unwired: 3 in]
    n134 = Index Array(array=w222, index=24) -> (element=→"Robot mode":u8)
    n135 = Array Subset(array=w222, index=16, length=8) -> (→"DigitalOutput":u8[])
    n136 = Array Subset(array=w222, index=664, length=8) -> (w235:u8[])
    n137 = Array Subset(array=w222, index=640, length=8) -> (w251:u8[])
    n138 = Array Subset(array=w222, index=648, length=8) -> (w249:u8[])
    n139 = Array Subset(array=w222, index=656, length=8) -> (w247:u8[])
    n140 = Array Subset(array=w222, index=632, length=8) -> (w252:u8[])
    n141 = Array Subset(array=w222, index=624, length=8) -> (w239:u8[])
    n142 = Reverse 1D Array(array=w235) -> (reversed array=w234:u8[])
    n143 = Reverse 1D Array(array=w247) -> (reversed array=w246:u8[])
    n144 = Reverse 1D Array(array=w251) -> (reversed array=w250:u8[])
    n145 = Reverse 1D Array(array=w239) -> (reversed array=w238:u8[])
    n146 = Reverse 1D Array(array=w252) -> (reversed array=w253:u8[])
    n147 = Reverse 1D Array(array=w249) -> (reversed array=w248:u8[])
    n148 = Type Cast(type=0.0, x=w234) -> (*(type *) &x=w254:dbl)
    n149 = Type Cast(type=0.0, x=w246) -> (*(type *) &x=w258:dbl)
    n150 = Type Cast(type=0.0, x=w250) -> (*(type *) &x=w266:dbl)
    n151 = Type Cast(type=0.0, x=w253) -> (*(type *) &x=w270:dbl)
    n152 = Type Cast(type=0.0, x=w248) -> (*(type *) &x=w262:dbl)
    n153 = Type Cast(type=0.0, x=w238) -> (*(type *) &x=w274:dbl)
    n154 = Array Subset(array=w222, index=64, length=8) -> (w229:u8[])
    n155 = Number To Fractional String(number=w254) -> (F-format string=→"rz value":string)  [unwired: 3 in]
    n156 = Number To Fractional String(number=w266) -> (F-format string=→"z value":string)  [unwired: 3 in]
    n157 = Number To Fractional String(number=w262) -> (F-format string=→"rx value":string)  [unwired: 3 in]
    n158 = Number To Fractional String(number=w258) -> (F-format string=→"ry value":string)  [unwired: 3 in]
    n159 = Number To Fractional String(number=w270) -> (F-format string=→"y value":string)  [unwired: 3 in]
    n160 = Number To Fractional String(number=w274) -> (F-format string=→"x value":string)  [unwired: 3 in]
    n161 = Reverse 1D Array(array=w229) -> (reversed array=w228:u8[])
    n162 = Type Cast(type=0.0, x=w228) -> (*(type *) &x=→"Current SpeedFactor":dbl)
    n163 = Or(x=w320, y=w318) -> (x .or. y?=w319:bool)
  }
  n164 = TCP Close Connection(connection ID=w10) -> ()  [unwired: 2 in, 2 out]
  n165 = TCP Close Connection(connection ID=w9) -> ()  [unwired: 2 in, 2 out]
